vi "Run greeter_client.vi"(10 "Request Data":T2={"name"="John"}) -> (0 "error out":errorcluster, 3 "Response Data":T1)   [LabVIEW 2019, in "helloworld_client.lvlib"]
uses:
  helloworld_client.lvlib
  RPC Messages/helloworld_HelloRequest.ctl
  RPC Messages/helloworld_HelloReply.ctl
panel:
  in  "error in":errorcluster
  in  "Server Address":string="localhost:50051"
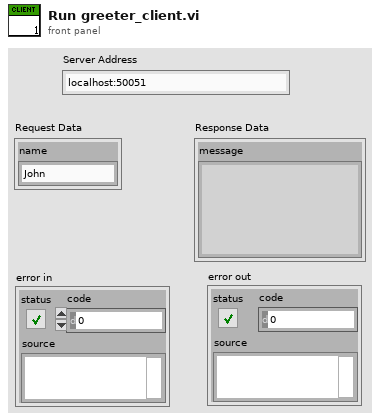
[diagram p1: front panel]
types:
  T1 = typedef "helloworld_client.lvlib/helloworld_HelloReply.ctl" = cluster{"message":string}
  T2 = typedef "helloworld_client.lvlib/helloworld_HelloRequest.ctl" = cluster{"name":string}
  T3 = typedef "grpc-lvsupport-release.lvlib/grpcId.ctl" = u64
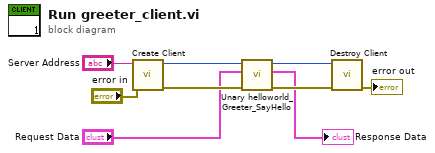
[diagram p0: block diagram]
diagram:
  n1 = call "Create Client.vi"("error in"="error in", "address"="Server Address") -> ("error out"=w7:errorcluster, "gRPC ID Out"=w8:T3)  [unwired: 8 in]
  n2 = call "Unary helloworld_Greeter_SayHello.vi"("error in"=w7, "Request Data"="Request Data", "gRPC ID"=w8) -> ("error out"=w6:errorcluster, "Response Data"=→"Response Data":T1, "gRPC ID out"=w5:T3)  [unwired: 6 in]
  n3 = call "Destroy Client.vi"("error in"=w6, "gRPC ID"=w5) -> ("error out"=→"error out":errorcluster)  [unwired: 9 in]
